vi "setIpAddress.vi"(8 "error":errorcluster, 10 "address":string, 11 "connection ID":refnum<k5>) -> (0 "error out":errorcluster, 3 "connection ID out":refnum<k5>)   [LabVIEW 2016, in "sen_api.lvlib"]
doc: "Sets the IP address of the device."
uses:
  sen_api.lvlib
panel:
  out "jsonRespIn":string
  out "JSON-response":string="{\"jsonrpc\":\"2.0\",\"method\":\"\",\"params\":[5,1.245,true,\"name\"],\"id\":\"1\"}"
  out "JSON request":string
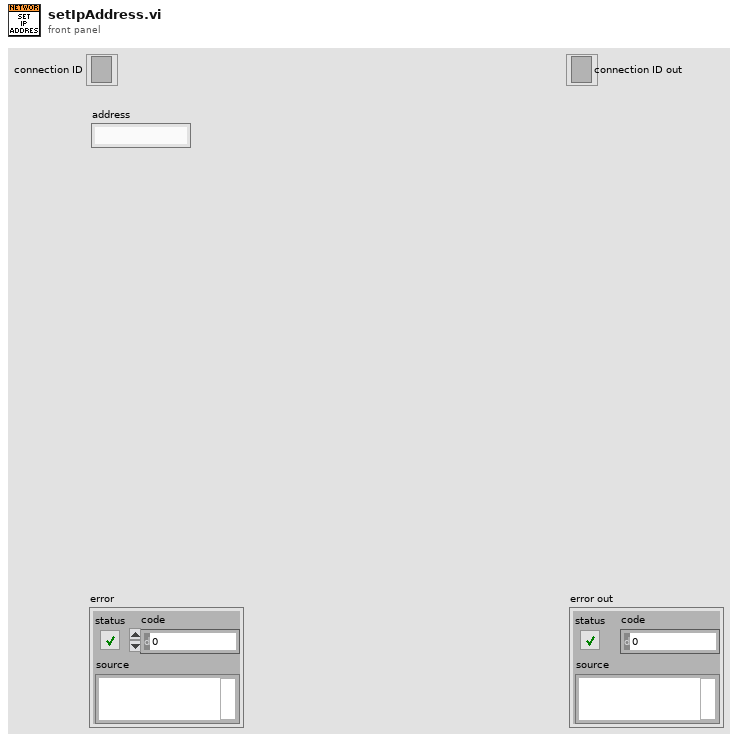
[diagram p1: front panel]
types:
  T1 = cluster{"jsonrpc":string, "method":string, "params":string[], "id":string, "api":i32, "pid":string}
  T2 = enum16{"Standard", "Buffered", "CRLF", "Immediate"}
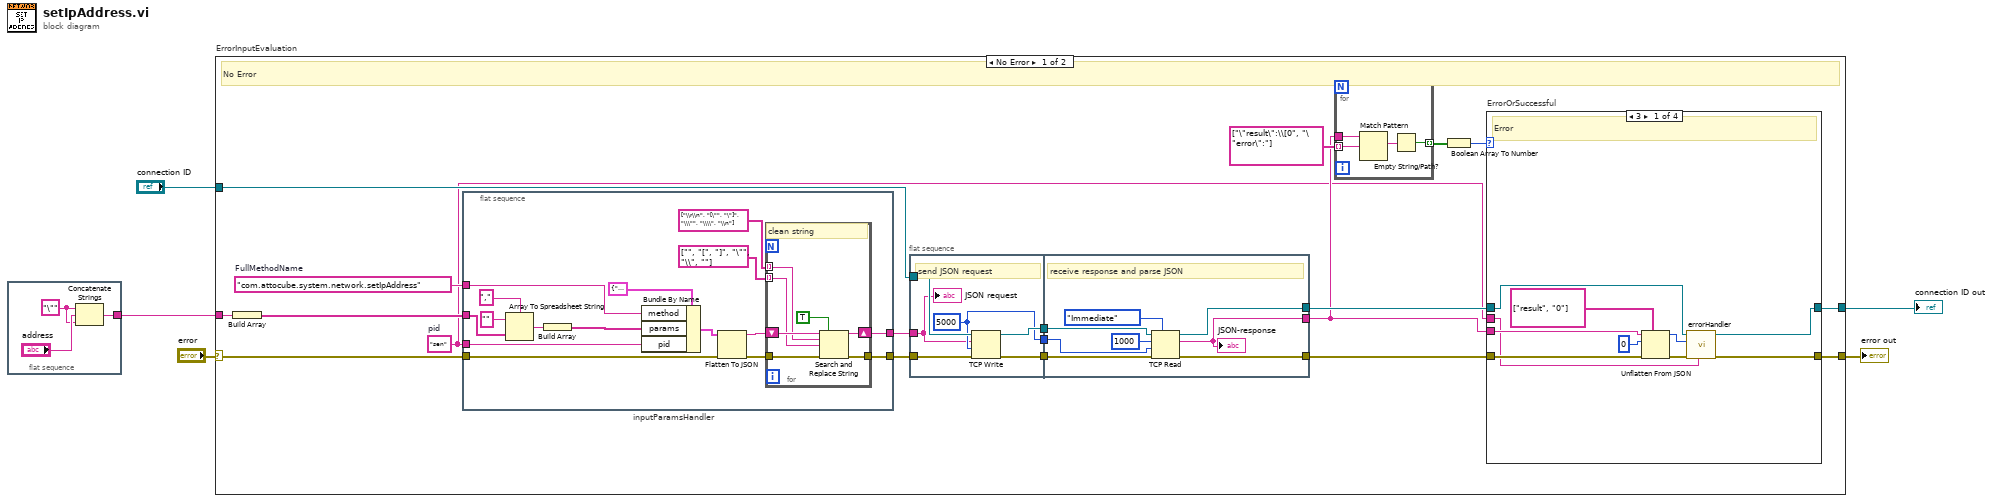
[diagram p0: block diagram]
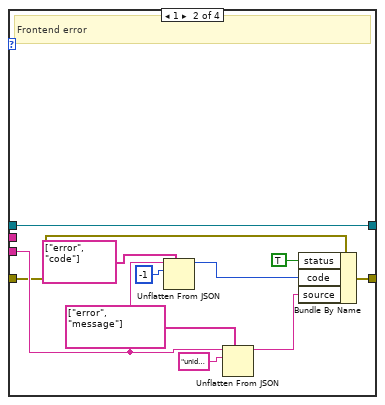
[diagram p2: hidden frame]
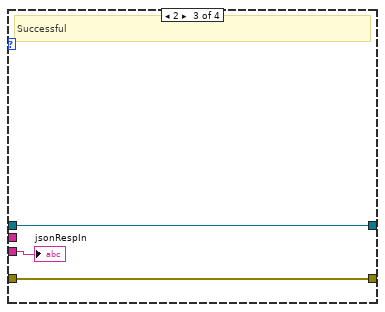
[diagram p3: hidden frame]
diagram:
  n1 = flat-sequence "in_string" {
    tunnel: [w7] -> w1
    frame #0 {
      w6 = "\"" ("string")
      n2 = Concatenate Strings(w6, "address", w6) -> (w7:string)
    }
  }
  n3 = case "ErrorInputEvaluation" shown="No Error" "error" {
    selector: "error" -> [w14 w95]
    tunnel: "connection ID" -> [w24 w96]
    tunnel: [w16 w95] -> w4
    tunnel: [w17 w96] -> w3
    tunnel: w1 -> [w9 _]
    frame No Error {
      w10 = "sen"  # pid
      w15 = "com.attocube.system.network.setIpAddress"  # FullMethodName
      # "No Error"
      n4 = Build Array ("ParametersArrayString")(w9) -> (w13:string[])
      n5 = flat-sequence "inputParamsHandler" {
        tunnel: [w31] -> w12
        tunnel: w13 -> [w38]
        tunnel: w14 -> [w36]
        tunnel: [w33] -> w11
        tunnel: w15 -> [w39]
        tunnel: w10 -> [w28]
        frame #0 {
          n6 = Array To Spreadsheet String(delimiter (Tab)=",", array=w38, 3:"" ("format string")) -> (spreadsheet string=w41:string)
          n7 = Build Array "Build Array"(w41) -> (w37:string[])
          n8 = Bundle By Name(cluster=T1 {"jsonrpc"="2.0", "method"="com.attocube.amc.res.setRESReadOutFreq", "params"=[], "id"="1", "api"=2, "pid"=""}, "method"=w39, "params"=w37, "pid"=w28) -> (w40:T1)
          n9 = Flatten To JSON(anything=w40, error in (no error)=w36) -> (JSON string=w32:string, 11:w34:errorcluster)  [unwired: 1 in]
          n10 = for {
            tunnel: string[] ["\\r\\n", "[\"", "\"]", "\\\"", "\\\\", "\\n"] ("search string") -> [w47] mode=indexing
            tunnel: string[] ["", "[", "]", "\"", "\\", ""] ("replace string (\"\")") -> [w46] mode=indexing
            shift-right: [w49] -> w31
            shift-left: w32 -> [w48]
            tunnel: w34 -> [w45]
            tunnel: [w44] -> w33
            # "clean string"
            n11 = Search and Replace String(replace all?=TRUE ("replace all? (F)"), input string=w48, search string=w47, replace string=w46, error in=w45) -> (result string=w49:string, error out=w44:errorcluster)  [unwired: 3 in, 2 out]
          }
        }
      }
      n12 = flat-sequence {
        tunnel: w24 -> [w86]
        tunnel: [w84] -> w27
        tunnel: [w85] -> w26
        tunnel: w11 -> [w81]
        tunnel: [w83] -> w25
        tunnel: w12 -> [w82]
        tunnel: [w90] -> w20
        tunnel: w27 -> [w92]
        tunnel: w26 -> [w91]
        tunnel: [w88] -> w19
        tunnel: w25 -> [w89]
        tunnel: [w87] -> w18
        frame #0 {
          w83 = 5000 ("timeout ms (25000)")
          # "send JSON request"
          n13 = TCP Write(connection ID=w86, data in=w82, error in (no error)=w81, 9:w83) -> (connection ID out=w84:refnum<k5>, error out=w85:errorcluster)  [unwired: 1 out]
          "JSON request" <- w82
        }
        frame #1 {
          # "receive response and parse JSON"
          n14 = TCP Read(connection ID=w92, bytes to read=1000, error in (no error)=w91, 7:T2."Immediate" ("mode (standard)"), 9:w89) -> (connection ID out=w90:refnum<k5>, data out=w87:string, error out=w88:errorcluster)
          "JSON-response" <- w87
        }
      }
      n15 = for {
        tunnel: string[] ["\"result\":\\[0", "\"error\":"] ("path") -> [w53] mode=indexing
        tunnel: [w51] -> w22 mode=indexing
        tunnel: w18 -> [w54]
        n16 = Match Pattern(string=w54, regular expression=w53) -> (match substring=w52:string)  [unwired: 1 in, 3 out]
        n17 = Empty String/Path?(string/path=w52) -> (empty?=w51:bool)
      }
      n18 = Boolean Array To Number(Boolean array=w22) -> (number=w21:u32)
      n19 = case "ErrorOrSuccessful" shown="3" w21 {
        tunnel: w18 -> [w58 w67 w76 _]
        tunnel: w20 -> [w62 w65 w78 w80]
        tunnel: [w60 w65 w78 w80] -> w17
        tunnel: [w61 w68 w77 w79] -> w16
        tunnel: w19 -> [w64 w66 w77 w79]
        tunnel: w10 -> [w55 _ _ _]
        frame 3 {
          # "Error"
          n20 = Unflatten From JSON(path=string[] ["result", "0"], JSON string=w58, type and defaults=0, error in (no error)=w64) -> (value=w56:i32, error out=w63:errorcluster)  [unwired: 3 in]
          n21 = call "errorHandler.vi"("pid"=w55, "error in"=w63, "errNbr"=w56, "connection ID"=w62) -> ("error out 2"=w61:errorcluster, "connection ID out"=w60:refnum<k5>)  [unwired: 6 in]
        }
        frame 1 {
          # "Frontend error"
          n22 = Unflatten From JSON(path=string[] ["error", "code"], JSON string=w67, type and defaults=-1) -> (value=w74:i32)  [unwired: 4 in, 1 out]
          n23 = Unflatten From JSON(path=string[] ["error", "message"], JSON string=w67, type and defaults="unidentified error") -> (value=w75:string)  [unwired: 4 in, 1 out]
          n24 = Bundle By Name(cluster=w66, "status"=TRUE, "code"=w74, "source"=w75) -> (w68:errorcluster)
        }
        frame 2 {
          # "Successful"
          "jsonRespIn" <- w76
        }
        frame Default {
          # "NoResponse"
        }
      }
    }
    frame Error {
      # "Error"
    }
  }
  "error out" <- w4
  "connection ID out" <- w3
